vi "LEDStateController.vi"(1 "Selected State (In)":string) -> (0 "Selected State (Out)":string)   [LabVIEW 2019]
doc: "This VI manages the apperance of the decorative LEDs. The LED coloration and blink pattern report the robot mode and status. See project documentation for details."
uses:
  outputs.vi
  dsdata.vi
  dsinstructions.vi
panel:
  in  "Diverting Power":dbl(slide)=0.99 min=-1.0 max=1.0 scale=-1.0..1.0
  in  "Human Player Signal":dbl(slide)=-0.89 min=-1.0 max=1.0 scale=-1.0..1.0
  in  "Master Caution":dbl(slide)=0.61 min=-1.0 max=1.0 scale=-1.0..1.0
  in  "Robot Oriented":dbl(slide)=0.57 min=-1.0 max=1.0 scale=-1.0..1.0
  in  "Field Oriented":dbl(slide)=0.85 min=-1.0 max=1.0 scale=-1.0..1.0
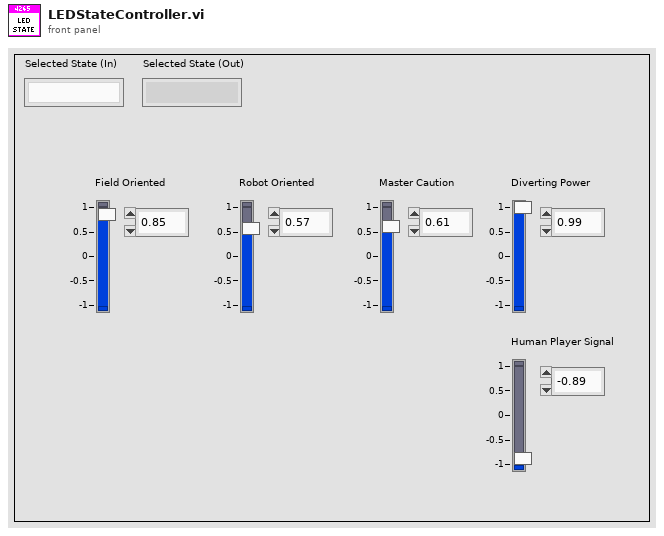
[diagram p1: front panel]
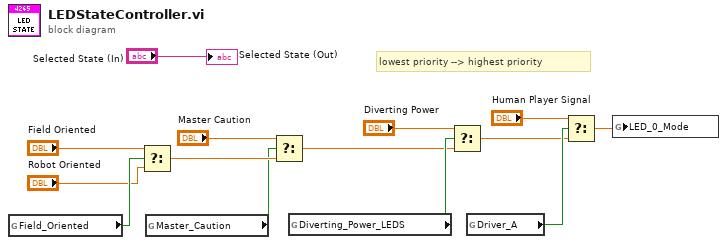
[diagram p0: block diagram]
diagram:
  # "lowest priority --> highest priority"
  n1 = global read "outputs.vi" "Field_Oriented"() -> (w13:bool)
  n2 = Select(t="Field Oriented", s=w13, f="Robot Oriented") -> (s? t:f=w10:dbl)
  n3 = global read "dsdata.vi" "Master_Caution"() -> (w9:bool)
  n4 = Select(t="Master Caution", s=w9, f=w10) -> (s? t:f=w1:dbl)
  n5 = global read "outputs.vi" "Diverting_Power_LEDS"() -> (w3:bool)
  n6 = Select(t="Diverting Power", s=w3, f=w1) -> (s? t:f=w4:dbl)
  n7 = global read "dsinstructions.vi" "Driver_A"() -> (w5:bool)
  n8 = Select(t="Human Player Signal", s=w5, f=w4) -> (s? t:f=w6:dbl)
  n9 = global write "outputs.vi" "LED_0_Mode"(w6) -> ()
  "Selected State (Out)" <- "Selected State (In)"
